vi "Constructor.vi"(0 "Core In":refnum<class "Core.lvclass">, 11 "Error In":errorcluster {"Code" format="%.0x"}) -> (4 "Core Out":refnum<class "Core.lvclass">, 15 "Error Out":errorcluster {"Code" format="%.0x"})   [LabVIEW 2020, in "Core.lvlib" / "Core.lvclass"]
doc: "Constructor of a new object instance of this class."
uses:
  Core.lvclass
  Core.lvclass/Core.ctl
  Data.ctl
  Build.ctl
  SetCore.vi
  SetInstance.vi
panel:
  # "/* Locals */"
  # "/* Inputs */"
  # "/* Outputs */"
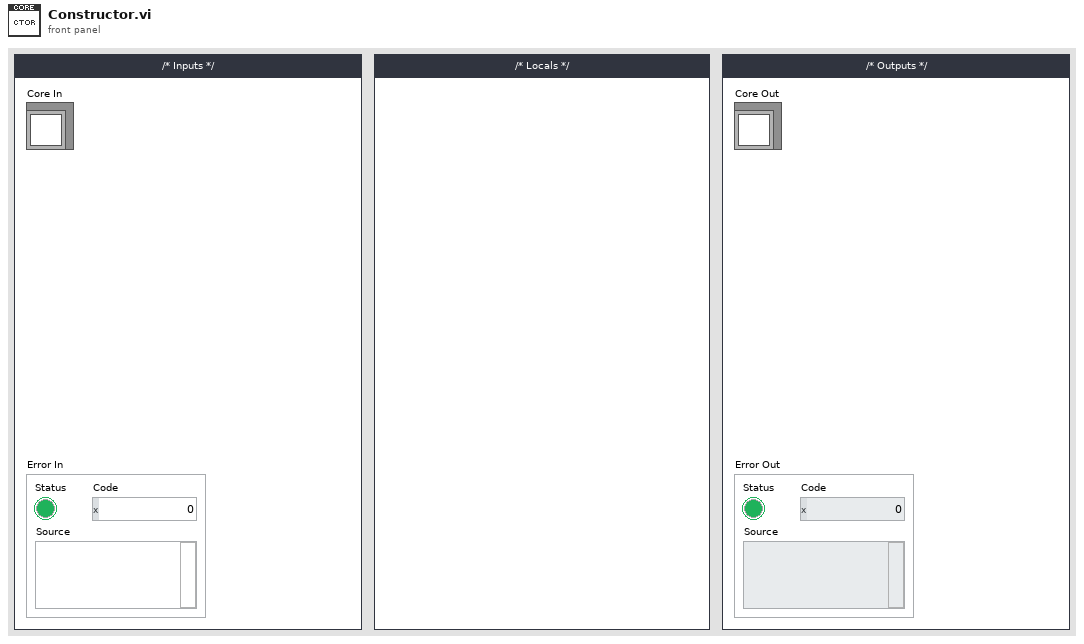
[diagram p1: front panel]
types:
  T1 = typedef "Core.lvlib/Core.lvclass/Data.ctl" = cluster{"Core":refnum<class "Core.lvclass">, "Instance":refnum<vi>, "Name":string, "Namespace":string, "Build":T2}
  T2 = typedef "Core.lvlib/Core.lvclass/Build.ctl" = cluster{"Computer":string, "PlatformOS":string, "PlatformVer":string, "Timestamp":string, "Version":string, "Author":string, "Company":string, "GUID":string}
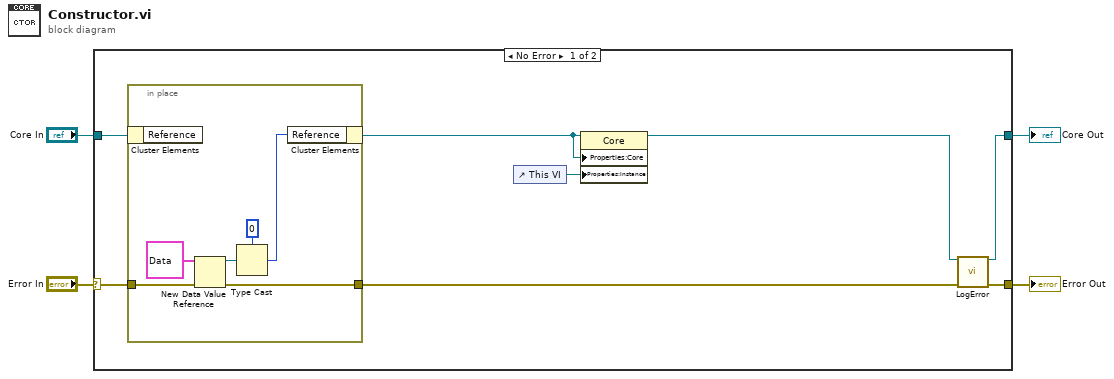
[diagram p0: block diagram]
diagram:
  n1 = case shown="No Error" "Error In" {
    selector: "Error In" -> [w12 w19]
    tunnel: [w9 w19] -> w3
    tunnel: "Core In" -> [w11 w20]
    tunnel: [w8 w20] -> w1
    frame No Error {
      n2 = in-place {
        in-place-border: w12 -> [w18]
        in-place-border: [w17] -> w10
        n3 = in-place-cluster #1(w11) -> ()  [unwired: 1 out]
        n4 = New Data Value Reference(data value=T1 {"Core"=refnum, "Instance"=refnum, "Name"="", "Namespace"="", "Build"={"Computer"="", "PlatformOS"="", "PlatformVer"="", "Timestamp"="", "Version"="", "Author"="", "Company"="", "GUID"=""}} ("Data"), error in=w18) -> (data value reference=w16:refnum<data-value>, error out=w17:errorcluster)
        n5 = Type Cast(type=u64 0, x=w16) -> (*(type *) &x=w14:u64)
        n6 = in-place-cluster #1("Reference"=w14) -> (w6:refnum<class "Core.lvclass">)
      }
      n7 = control-ref of="This VI"() -> (w5:refnum<vi>)
      n8 = property class="Core"(reference=w6, "Properties:Core"=w6, "Properties:Instance"=w5) -> (reference out=w7:refnum<class "Core.lvclass">)  [unwired: 1 in, 1 out]
      n9 = call-dynamic "LogError.vi"("Core In"=w7, "Error In"=w10) -> ("Core Out"=w8:refnum<class "Core.lvclass">, "Error Out"=w9:errorcluster)  [unwired: 12 in]
    }
    frame Error {
    }
  }
  "Core Out" <- w1
  "Error Out" <- w3
